vi "Check Input Duplicate.vi"(0 "Input Array":u8[][](array[numeric]), 7 "New Point":u8[](array[numeric])) -> (8 "Duplicate?":bool)   [LabVIEW 2010]
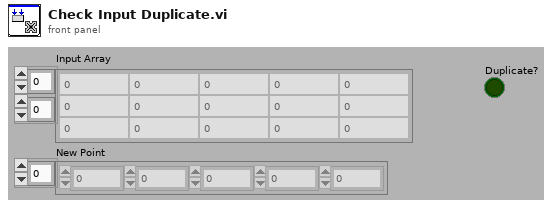
[diagram p1: front panel]
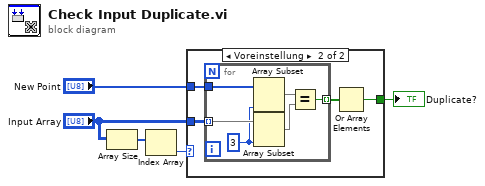
[diagram p0: block diagram]
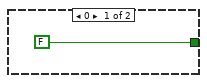
[diagram p2: hidden frame]
diagram:
  n1 = Array Size(array="Input Array") -> (size(s)=w2:i32[])
  n2 = Index Array(array=w2) -> (element=w1:i32)  [unwired: 1 in]
  n3 = case shown="Voreinstellung" w1 {
    tunnel: "New Point" -> [_ w9]
    tunnel: [FALSE w7] -> w4
    tunnel: "Input Array" -> [_ w10]
    frame 0 {
    }
    frame Default {
      n4 = for {
        tunnel: w10 -> [w14] mode=indexing
        tunnel: w9 -> [w16]
        tunnel: [w15] -> w8 mode=indexing
        w13 = 3 ("length")
        n5 = Array Subset(array=w16, length=w13) -> (w12:u8[])  [unwired: 1 in]
        n6 = Array Subset(array=w14, length=w13) -> (w11:u8[])  [unwired: 1 in]
        n7 = Equal?(x=w12, y=w11) -> (x = y?=w15:bool)
      }
      n8 = Or Array Elements(Boolean array=w8) -> (logical OR=w7:bool)
    }
  }
  "Duplicate?" <- w4
